vi "Non Delay Scheduler Engine.vi"(8 "Number of  Jobs":i32=4, 9 "Number of Machines":i32=4, 10 "Processing Times":u16[][](array[numeric])=[[34, 15, 38, 95], [2, 89, 19, 7], [54, 70, 28, 34], [61, 9, 87, 29]], 11 "Schedule":u16[](array[numeric])=[12, 0, 7, 2, 6, 3, 13, 5, 1, 4, 14, 11, 10, 15, 8, 9]) -> (0 "Scheduled Jobs Order":u16[](array[numeric]), 1 "Job Completion Times":u16[](array[numeric]), 2 "Completion Times":u16[][](array[numeric]), 3 "Start Times":u16[][](array[numeric]), 4 "Machine Completion Times":u16[](array[numeric]))   [LabVIEW 2013, in "GanntChart.lvclass"]
uses:
  GanntChart.lvclass
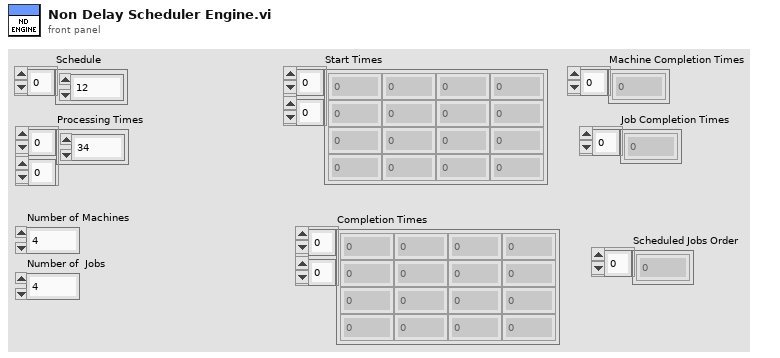
[diagram p1: front panel]
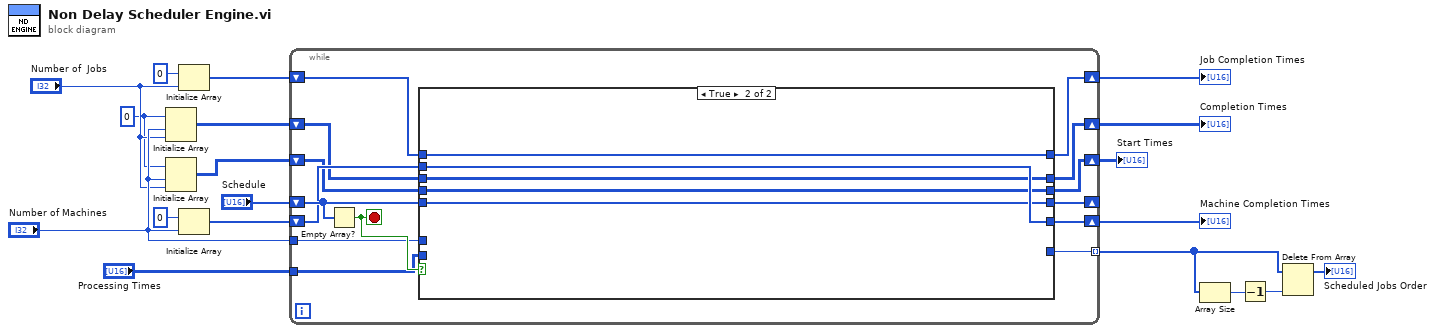
[diagram p0: block diagram]
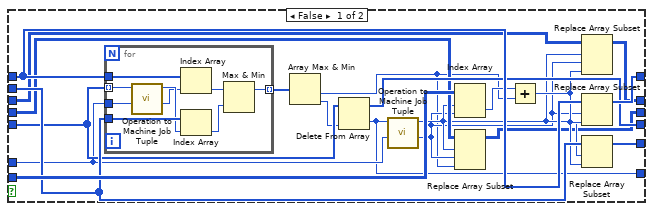
[diagram p2: hidden frame]
diagram:
  w3 = u16 0 ("element")
  n1 = Initialize Array(w3, "Number of Machines", "Number of  Jobs") -> (w14:u16[][])
  n2 = Initialize Array(w3, "Number of Machines", "Number of  Jobs") -> (w2:u16[][])
  n3 = Initialize Array(u16 0 ("element"), "Number of  Jobs") -> (w17:u16[])
  n4 = Initialize Array(u16 0 ("element"), "Number of Machines") -> (w16:u16[])
  n5 = while {
    shift-right: [w25] -> _
    shift-left: "Schedule" -> [w32]
    tunnel: "Number of Machines" -> [w31]
    shift-right: [w28] -> w12
    shift-left: w17 -> [w30]
    shift-right: [w27] -> w11
    shift-left: w16 -> [w29]
    shift-right: [w23] -> w13
    shift-left: w14 -> [w24]
    tunnel: "Processing Times" -> [w26]
    tunnel: [w22] -> w9 mode=indexing
    shift-right: [w20] -> w1
    shift-left: w2 -> [w21]
    stop <- w33 stop-if-true
    n6 = Empty Array?(array=w32) -> (empty?=w33:bool)
    n7 = case shown="True" w33 {
      tunnel: w32 -> [w45 w65]
      tunnel: w31 -> [w40 _]
      tunnel: w30 -> [w51 w67]
      tunnel: w29 -> [w52 w66]
      tunnel: [w50 w67] -> w28
      tunnel: [w49 w66] -> w27
      tunnel: w26 -> [w53 _]
      tunnel: [w44 w65] -> w25
      tunnel: w24 -> [w48 w64]
      tunnel: [w47 w64] -> w23
      tunnel: [w39 _] -> w22
      tunnel: w21 -> [w38 w63]
      tunnel: [w34 w63] -> w20
      frame False {
        n8 = for {
          tunnel: w45 -> [w62] mode=indexing
          tunnel: w40 -> [w61]
          tunnel: w51 -> [w58]
          tunnel: w52 -> [w60]
          tunnel: [w54] -> w46 mode=indexing
          n9 = call "Operation to Machine Job Tuple.vi"("Number of Machines"=w61, "Operation Number"=w62) -> ("Job No"=w57:i32, "Machine No"=w59:i32)  [unwired: 8 in]
          n10 = Index Array(array=w58, index=w57) -> (element=w56:u16)
          n11 = Index Array(array=w60, index=w59) -> (element=w55:u16)
          n12 = Max & Min(x=w56, y=w55) -> (max(x,y)=w54:u16)  [unwired: 1 out]
        }
        n13 = Array Max & Min(array=w46) -> (min value=w35:u16, min index (indices)=w41:i32)  [unwired: 2 out]
        n14 = Delete From Array(array=w45, index=w41) -> (deleted portion=w39:u16, array with subset deleted=w44:u16[])  [unwired: 1 in]
        n15 = call "Operation to Machine Job Tuple.vi"("Number of Machines"=w40, "Operation Number"=w39) -> ("Job No"=w36:i32, "Machine No"=w37:i32)  [unwired: 8 in]
        n16 = Index Array(array=w53, index (row)=w37, index (col)=w36) -> (element=w43:u16)
        n17 = Replace Array Subset(array=w38, new element=w35, index (row)=w37, index (col)=w36) -> (w34:u16[][])
        n18 = Add(x=w43, y=w35) -> (x+y=w42:u16)
        n19 = Replace Array Subset(array=w48, new element=w42, index (row)=w37, index (col)=w36) -> (w47:u16[][])
        n20 = Replace Array Subset(array=w51, new element=w42, index=w36) -> (w50:u16[])
        n21 = Replace Array Subset(array=w52, new element=w42, index=w37) -> (w49:u16[])
      }
      frame True {
      }
    }
  }
  "Completion Times" <- w13
  "Job Completion Times" <- w12
  "Machine Completion Times" <- w11
  "Start Times" <- w1
  n22 = Array Size(array=w9) -> (size(s)=w8:i32)
  n23 = Decrement(x=w8) -> (x-1=w7:i32)
  n24 = Delete From Array(array=w9, index=w7) -> (array with subset deleted=→"Scheduled Jobs Order":u16[])  [unwired: 1 in, 1 out]
